vi "Error.vi"(8 "Data":string, 9 "?":T1) -> (0 "error out":errorcluster)   [LabVIEW 2016, in "JSON Value.lvclass"]
uses:
  JSON Data Classes/JSON Helper/JSON Value.lvclass
  Errors.ctl
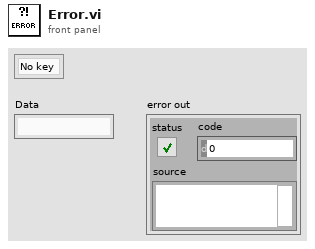
[diagram p1: front panel]
types:
  T1 = typedef "JSON Value.lvclass/Errors.ctl" = enum16{"No key", "Key path type", "Array OOB", "Type Mismatch", "Invalid Token"}
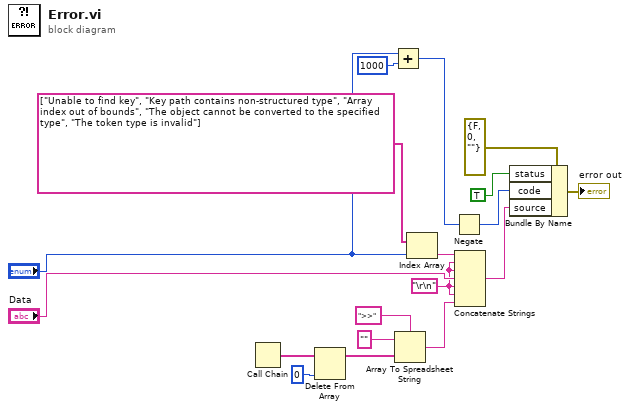
[diagram p0: block diagram]
diagram:
  w4 = "\r\n"
  n1 = Call Chain() -> (call chain=w16:string[])
  n2 = Delete From Array(array=w16, index=0) -> (array with subset deleted=w17:string[])  [unwired: 1 in, 1 out]
  n3 = Add(x="?", y=1000) -> (x+y=w12:i32)
  n4 = Array To Spreadsheet String(delimiter (Tab)=">>", array=w17, 3:"" ("format string")) -> (spreadsheet string=w3:string)
  n5 = Index Array(array=string[] ["Unable to find key", "Key path contains non-structured type", "Array index out of bounds", "The object cannot be converted to the specified type", "The token type is invalid"] ("[user-defined descriptions]"), index="?") -> (element=w6:string)
  n6 = Negate(x=w12) -> (-x=w9:i32)
  n7 = Concatenate Strings(w6, w4, w4, "Data", w4, w4, w3) -> (w2:string)
  n8 = Bundle By Name(cluster=errorcluster {"status"=FALSE, "code"=0, "source"=""} ("error out"), "status"=TRUE, "code"=w9, "source"=w2) -> (→"error out":errorcluster)
